vi "Lambda Calc.vi"(11 "Mexa In":dbl[](array[numeric])) -> (3 "Lambda Value":dbl)   [LabVIEW 2014]
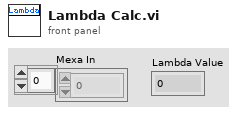
[diagram p1: front panel]
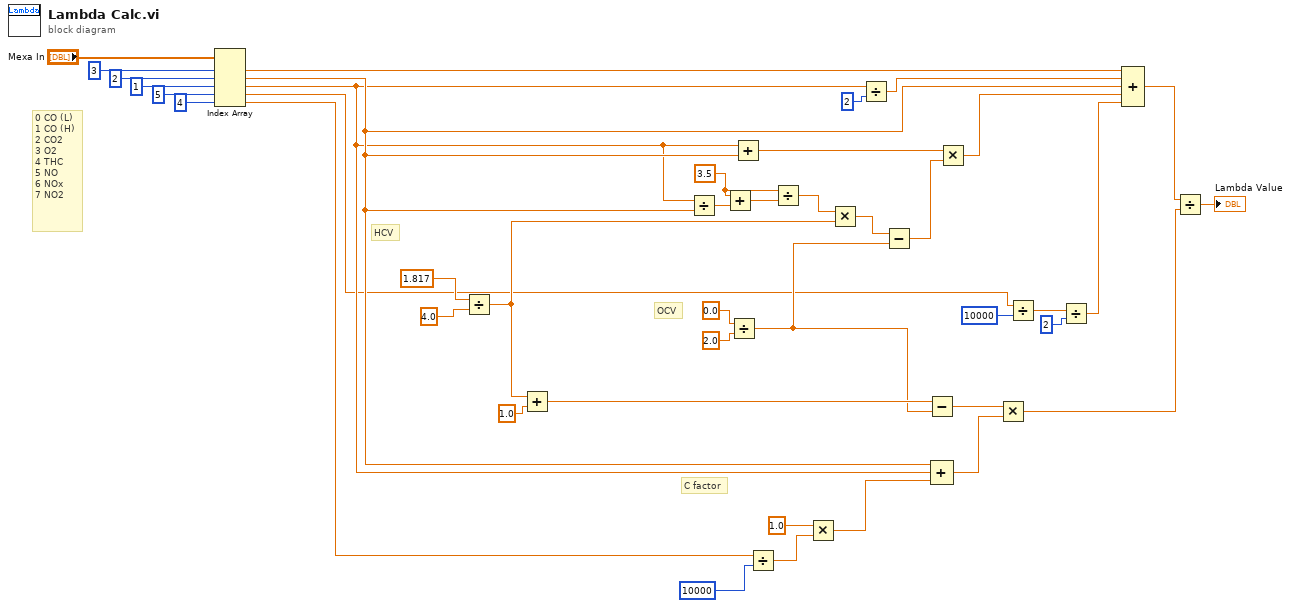
[diagram p0: block diagram]
diagram:
  w18 = 3.5
  # "0 CO (L)\n1 CO (H)\n2 CO2\n3 O2\n4 THC\n5 NO\n6 NOx\n7 NO2"
  # "C factor"
  # "OCV"
  # "HCV"
  n1 = Index Array(array="Mexa In", index #1=3 ("index"), index #2=2 ("index"), index #3=1 ("index"), index #4=5 ("index"), index #5=4 ("index")) -> (element #1=w10:dbl, element #2=w7:dbl, element #3=w6:dbl, element #4=w4:dbl, element #5=w2:dbl)
  n2 = Divide(x=1.817, y=4.0) -> (x/y=w14:dbl)
  n3 = Add(x=w14, y=1.0) -> (x+y=w35:dbl)
  n4 = Divide(x=w6, y=w7) -> (x/y=w17:dbl)
  n5 = Add(x=w18, y=w17) -> (x+y=w19:dbl)
  n6 = Divide(x=0.0, y=2.0) -> (x/y=w15:dbl)
  n7 = Add(x=w6, y=w7) -> (x+y=w21:dbl)
  n8 = Divide(x=w2, y=10000) -> (x/y=w34:dbl)
  n9 = Divide(x=w18, y=w19) -> (x/y=w16:dbl)
  n10 = Multiply(x=1.0, y=w34) -> (x*y=w32:dbl)
  n11 = Multiply(x=w16, y=w14) -> (x*y=w20:dbl)
  n12 = Divide(x=w6, y=2) -> (x/y=w26:dbl)
  n13 = Subtract(x=w20, y=w15) -> (x-y=w22:dbl)
  n14 = Subtract(x=w35, y=w15) -> (x-y=w31:dbl)
  n15 = Compound Arithmetic op=ADD(w7, w6, w32) -> (w30:dbl)
  n16 = Multiply(x=w21, y=w22) -> (x*y=w12:dbl)
  n17 = Multiply(x=w31, y=w30) -> (x*y=w28:dbl)
  n18 = Divide(x=w4, y=10000) -> (x/y=w13:dbl)
  n19 = Divide(x=w13, y=2) -> (x/y=w23:dbl)
  n20 = Compound Arithmetic op=ADD(w10, w26, w7, w12, w23) -> (w25:dbl)
  n21 = Divide(x=w25, y=w28) -> (x/y=→"Lambda Value":dbl)
